vi "UpdateProjectInfo.vi"(6 "Target FPGA Personality":string, 7 "Device Code":u32, 8 "error in (no error)":errorcluster, 9 "Target Address":string="0.0.0.0", 10 "Target Name":string="myRIO Target", 11 "MetaDataObj in":refnum<class "MetaDataObj.lvclass">) -> (0 "error out":errorcluster, 3 "MetaDataObj out":refnum<class "MetaDataObj.lvclass">)   [LabVIEW 2021, in "myRIOMetaDataObj.lvclass"]
uses:
  myRIOMetaDataObj.lvclass
  <resource>/dialog/NewProjectWizard/MetaDataObj/MetaDataObj.lvclass
  p:/lvdist/win32/export/21.0/21.0.0f0/dist/resource/dialog/NewProjectWizard/MetaDataObj/MetaDataObj.lvclass
  myRIOMetaDataObj.lvclass/myRIOMetaDataObj.ctl
  Write Target FPGA Personality.vi
  <resource>/dialog/NewProjectWizard/MetaDataObj/Accessors/Write Project Path.vi
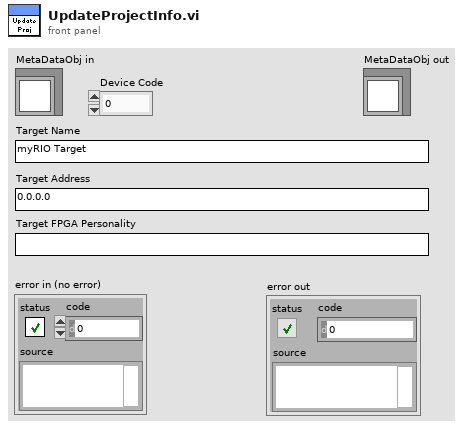
[diagram p1: front panel]
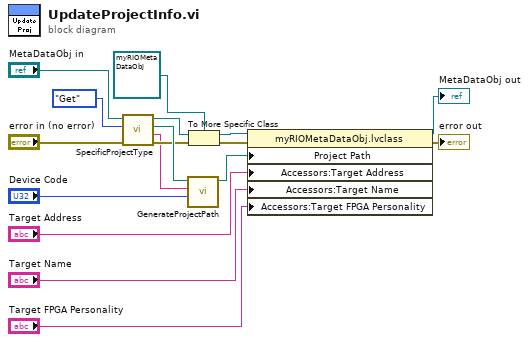
[diagram p0: block diagram]
diagram:
  n1 = call "SpecificProjectType.vi"("error in (no error)"="error in (no error)", "Action"=enum16{"Clear", "Get", "Set"}."Get", "MetaDataObj in"="MetaDataObj in") -> ("error out"=w8:errorcluster, "Project Name"=w2:string, "Project Root"=w12:path, "MetaDataObj out"=w9:refnum<class "MetaDataObj.lvclass">)  [unwired: 5 in]
  n2 = call "GenerateProjectPath.vi"("Device Code"="Device Code", "Project Name"=w2, "Location Path"=w12) -> ("Project Path"=w17:path)  [unwired: 8 in]
  n3 = To More Specific Class(target class=refnum<class "myRIOMetaDataObj.lvclass"> refnum ("myRIOMetaDataObj.lvclass"), reference=w9, error in=w8) -> (specific class reference=w6:refnum<class "myRIOMetaDataObj.lvclass">, error out=w7:errorcluster)
  n4 = property class="myRIOMetaDataObj.lvclass"(reference=w6, error in=w7, "Project Path"=w17, "Accessors:Target Address"="Target Address", "Accessors:Target Name"="Target Name", "Accessors:Target FPGA Personality"="Target FPGA Personality") -> (reference out=→"MetaDataObj out":refnum<class "myRIOMetaDataObj.lvclass">, error out=→"error out":errorcluster)
